vi "CCD LinePatternSetup v0.46.vi"(6 "CCD GPIB Address":u16=1, 9 "Shutter Enabled":bool=TRUE, 10 "Exposuretime (s)":dbl=0.5 format="%.2f") -> (2 "New Image Dimension":i32[](array[numeric]), 3 "Current Setup String":string="ldu,0,256,16;sdu,0,1024,1024;cl0;omrm;sron")   [LabVIEW 2020]
doc: "This VI sets up the CCD camera and assign the setup string to a global variable."
uses:
  Globals and TypeDefs/Global Varibal Control.vi
panel:
  in  "Show New Image":bool=TRUE caption="Show Full Image"
  in  "New Image shot":bool
  out "New Intensity graph":i32[][](graph)
  in  "CCD Lines":cluster{u8, u8}(slide)={0, 7} scale=1.0..256.0
  in  "Number of blocks":u8=25 min=1 max=25
  in  "pixel per block":u8=6 min=1 max=8
  out "#PixelOverflow":u32
  out "PixelOverflow":bool
  in  "Full Image Shot":bool
  in  "Set back to array":bool
  in  "Generate color table":bool
  in  "Stop button":bool
  out "Intensity graph":i32[][](graph)
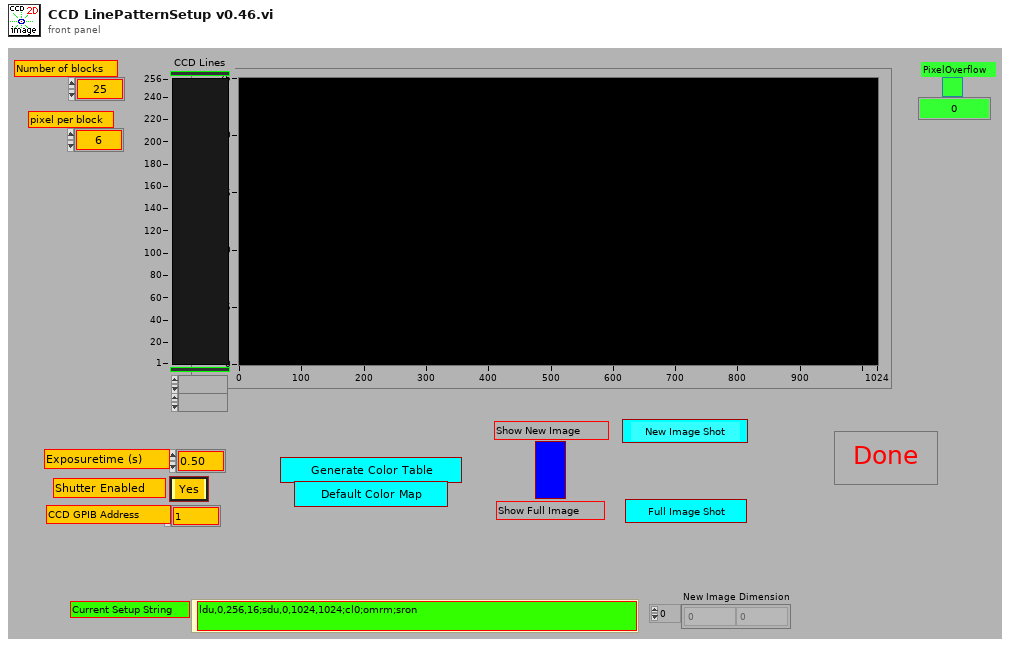
[diagram p1: front panel]
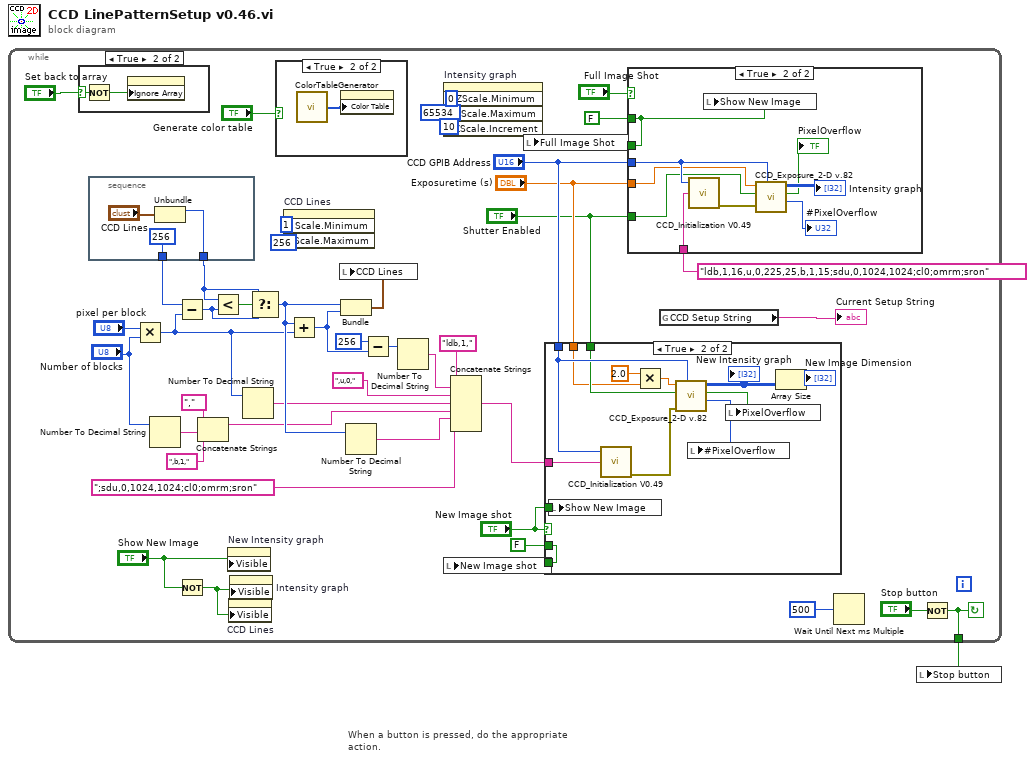
[diagram p0: block diagram]
diagram:
  n1 = while "When a button is pressed, do the appropriate action." {
    tunnel: [w40] -> w1
    stop <- w40 continue-if-true
    n2 = case shown="True" "Set back to array" {
      selector: "Set back to array" -> [_ w76]
      frame False {
      }
      frame True {
        n3 = Not(x=w76) -> (.not. x?=w75:bool)
        n4 = property class="IntGraph (strict)"("Ignore Array"=w75) -> ()  [unwired: 2 in, 2 out]
      }
    }
    n5 = stacked-sequence {
      tunnel: [u16 256 ("Maximum")] -> w34
      tunnel: [w63] -> w35
      frame #0 {
        n6 = Unbundle("CCD Lines") -> (w63:u8)  [unwired: 1 out]
      }
    }
    n7 = Multiply(x="pixel per block", y="Number of blocks") -> (x*y=w22:u8)
    n8 = Number To Decimal String(number="Number of blocks") -> (decimal integer string=w12:string)  [unwired: 1 in]
    n9 = Subtract(x=w34, y=w22) -> (x-y=w24:u16)
    n10 = Not(x="Show New Image") -> (.not. x?=w8:bool)
    n11 = Concatenate Strings(",", w12, ",b,1,") -> (w11:string)
    n12 = Less?(x=w35, y=w24) -> (x < y?=w25:bool)
    n13 = property on="New Intensity graph" class="IntGraph (strict)"("Visible"="Show New Image") -> ()  [unwired: 2 in, 2 out]
    n14 = property on="CCD Lines" class="Slide (strict)"("Visible"=w8) -> ()  [unwired: 2 in, 2 out]
    n15 = property on="Intensity graph" class="IntGraph (strict)"("Visible"=w8) -> ()  [unwired: 2 in, 2 out]
    n16 = Number To Decimal String(number=w22) -> (decimal integer string=w14:string)  [unwired: 1 in]
    n17 = Select(t=w35, s=w25, f=w24) -> (s? t:f=w23:u16)
    n18 = case shown="True" "Generate color table" {
      frame False {
      }
      frame True {
        n19 = call "ColorTableGenerator.vi"() -> (w77:u32[])
        n20 = property on="Intensity graph" class="IntGraph (strict)"("Color Table"=w77) -> ()  [unwired: 2 in, 2 out]
      }
    }
    n21 = property on="CCD Lines" class="Slide (strict)"("Scale.Minimum"=u8 1 ("Minimum"), "Scale.Maximum"=u16 256 ("Maximum")) -> ()  [unwired: 2 in, 2 out]
    n22 = Add(x=w23, y=w22) -> (x+y=w21:u16)
    n23 = Bundle(w23, w21) -> (w38:cluster{u16, u16})  [unwired: 1 in]
    n24 = local write "CCD Lines"(w38) -> ()
    n25 = Number To Decimal String(number=w23) -> (decimal integer string=w4:string)  [unwired: 1 in]
    n26 = Subtract(x=u16 256, y=w21) -> (x-y=w19:u16)
    n27 = Number To Decimal String(number=w19) -> (decimal integer string=w5:string)  [unwired: 1 in]
    n28 = property on="Intensity graph" class="IntGraph (strict)"("ZScale.Minimum"=u32 0 ("Z Minimum"), "ZScale.Maximum"=u32 65534 ("Z Maximum"), "ZScale.Increment"=u32 10 ("Z Increment")) -> ()  [unwired: 2 in, 2 out]
    n29 = Concatenate Strings("ldb,1,", w5, ",u,0,", w14, w11, w4, ";sdu,0,1024,1024;cl0;omrm;sron") -> (w3:string)
    n30 = case shown="True" "New Image shot" {
      tunnel: [w48 w55] -> w30
      tunnel: FALSE -> [w48 w55]
      tunnel: "CCD GPIB Address" -> [_ w61]
      tunnel: "Exposuretime (s)" -> [_ w52]
      tunnel: "Shutter Enabled" -> [_ w60]
      tunnel: w3 -> [_ w49]
      tunnel: "New Image shot" -> [_ w54]
      frame False {
      }
      frame True {
        n31 = local write "Show New Image"(w54) -> ()
        n32 = call "CCD_Initialization V0.49.vi"("Setup String"=w49, "CCD GPIB Address"=w61) -> ("error out"=w59:errorcluster)  [unwired: 3 in, 3 out]
        n33 = Multiply(x=2.0, y=w52) -> (x*y=w51:dbl)
        n34 = call "CCD_Exposure_2-D v.82.vi"("CCD GPIB Address"=w61, "error in"=w59, "Shutter Enabled"=w60, "Exposuretime (s)"=w51) -> ("#PixelOverflow"=w56:u32, "PixelOverflow"=w57:bool, "The Data"=w58:i32[][])  [unwired: 1 in, 4 out]
        "New Intensity graph" <- w58
        n35 = local write "#PixelOverflow"(w56) -> ()
        n36 = local write "PixelOverflow"(w57) -> ()
        n37 = Array Size(array=w58) -> (size(s)=→"New Image Dimension":i32[])
      }
    }
    n38 = local write "New Image shot"(w30) -> ()
    n39 = case shown="True" "Full Image Shot" {
      tunnel: "ldb,1,16,u,0,225,25,b,1,15;sdu,0,1024,1024;cl0;omrm;sron" -> [_ w66]
      tunnel: [w65 w67] -> w31
      tunnel: FALSE -> [w65 w67]
      tunnel: "CCD GPIB Address" -> [_ w70]
      tunnel: "Shutter Enabled" -> [_ w69]
      tunnel: "Exposuretime (s)" -> [_ w68]
      frame False {
      }
      frame True {
        n40 = call "CCD_Initialization V0.49.vi"("Setup String"=w66, "CCD GPIB Address"=w70) -> ("error out"=w71:errorcluster)  [unwired: 3 in, 3 out]
        n41 = local write "Show New Image"(w67) -> ()
        n42 = call "CCD_Exposure_2-D v.82.vi"("CCD GPIB Address"=w70, "error in"=w71, "Shutter Enabled"=w69, "Exposuretime (s)"=w68) -> ("#PixelOverflow"=→"#PixelOverflow":u32, "PixelOverflow"=→"PixelOverflow":bool, "The Data"=→"Intensity graph":i32[][])  [unwired: 1 in, 4 out]
      }
    }
    n43 = local write "Full Image Shot"(w31) -> ()
    n44 = global read "Global Varibal Control.vi" "CCD Setup String"() -> (→"Current Setup String":string)
    n45 = Wait Until Next ms Multiple(millisecond multiple=u32 500) -> ()  [unwired: 1 out]
    n46 = Not(x="Stop button") -> (.not. x?=w40:bool)
  }
  n47 = local write "Stop button"(w1) -> ()
